vi "TCPReadCmd.vi"(8 "error in (no error)":errorcluster, 9 "timeout ms (25000)":i32=25000, 10 "on timeout wait before close (500 ms)":u32=500, 11 "connection ID":refnum<k5>) -> (0 "error out":errorcluster, 2 "Command Code":string, 3 "connection ID out":refnum<k5>)   [LabVIEW 2013]
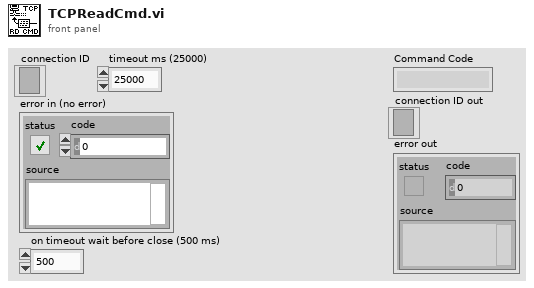
[diagram p1: front panel]
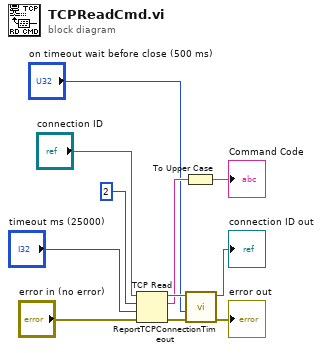
[diagram p0: block diagram]
diagram:
  n1 = TCP Read(connection ID="connection ID", bytes to read=2, error in (no error)="error in (no error)", 9:"timeout ms (25000)") -> (connection ID out=w9:refnum<k5>, data out=w8:string, error out=w10:errorcluster)  [unwired: 1 in]
  n2 = To Upper Case(1:w8) -> (0:→"Command Code":string)
  n3 = call "ReportTCPConnectionTimeout.vi"("error in (no error)"=w10, "wait before close (500 ms)"="on timeout wait before close (500 ms)", "connection ID"=w9) -> ("error out"=→"error out":errorcluster, "connection ID out"=→"connection ID out":refnum<k5>)  [unwired: 7 in]
